vi "RSZVB Get Generator Step Attenuators.vi"(8 "error in (no error)":errorcluster {"code" format="%.0x"}, 9 "Port (1)":i32=1, 10 "Channel (1)":i32=1, 11 "VISA session":refnum<visa-resource-name>) -> (0 "error out":errorcluster {"code" format="%.0x"}, 1 "Attenuation Factor":dbl format="%^.3e", 3 "dup VISA session":refnum<visa-resource-name>)   [LabVIEW 2011]
doc: "This VI gets a fixed attenuation factor for the generated wave at test port no. <Pt>. \n\nNote(s):\n\n(1) This VI can be used only with R&S ZVA and ZVB instruments.\n\nRemote-control command(s):\nSOURce<Ch>:POWer<Pt>:ATTenuation?"
uses:
  _utility/RSZVB Global Data.vi
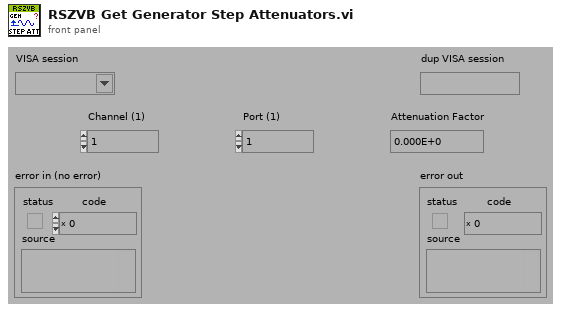
[diagram p1: front panel]
types:
  T1 = cluster{"Error Checking (T: On)":bool, "Installed Options":string[], "Data Valid?":bool, "Ports":i32, "Model":string[], "Option Checking (T: On)":bool}[]
  T2 = cluster{"Error Checking (T: On)":bool, "Installed Options":string[], "Data Valid?":bool, "Ports":i32, "Model":string[], "Option Checking (T: On)":bool}
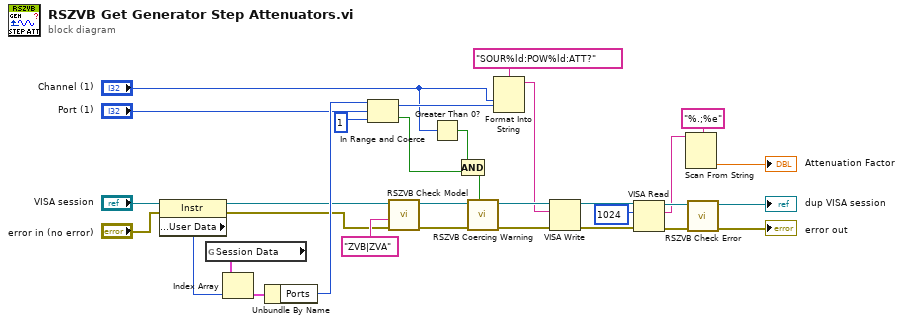
[diagram p0: block diagram]
diagram:
  n1 = property class="Instr"(reference="VISA session", error in="error in (no error)") -> (reference out=w19:refnum<visa-resource-name>, error out=w18:errorcluster, "General Settings:User Data"=w21:u32)
  n2 = global read "RSZVB Global Data.vi" "Session Data"() -> (w22:T1)
  n3 = Index Array(array=w22, index=w21) -> (element=w23:T2)
  n4 = Unbundle By Name(w23) -> ("Ports"=w20:i32)
  n5 = In Range and Coerce(upper limit=w20, x="Port (1)", lower limit=1) -> (coerced(x)=w16:i32, In Range?=w17:bool)
  n6 = call "RSZVB Check Model.vi"("error in (no error)"=w18, "Model"="ZVB|ZVA" ("Options"), "VISA session"=w19) -> ("error out"=w26:errorcluster, "dup VISA session"=w25:refnum<visa-resource-name>)  [unwired: 7 in]
  n7 = Greater Than 0?(x="Channel (1)") -> (x > 0?=w27:bool)
  n8 = Compound Arithmetic op=AND(w27, w17) -> (w29:bool)
  n9 = call "RSZVB Coercing Warning.vi"("In Range?"=w29, "error in (no error)"=w26, "VISA session"=w25) -> ("error out"=w30:errorcluster, "dup VISA session"=w31:refnum<visa-resource-name>)  [unwired: 7 in]
  n10 = Format Into String(format string="SOUR%ld:POW%ld:ATT?", "Channel (1)", w16) -> (resulting string=w28:string)  [unwired: 2 in, 1 out]
  n11 = VISA Write(VISA resource name=w31, write buffer=w28, error in (no error)=w30) -> (VISA resource name out=w5:refnum<visa-resource-name>, error out=w1:errorcluster)  [unwired: 1 out]
  n12 = VISA Read(VISA resource name=w5, byte count=u32 1024 ("byte count (0)"), error in (no error)=w1) -> (VISA resource name out=w9:refnum<visa-resource-name>, read buffer=w6:string, error out=w8:errorcluster)  [unwired: 1 out]
  n13 = Scan From String(format string="%.;%e", input string=w6) -> (output 1=→"Attenuation Factor":dbl)  [unwired: 3 in, 3 out]
  n14 = call "RSZVB Check Error.vi"("error in (no error)"=w8, "VISA session"=w9) -> ("error out"=→"error out":errorcluster, "dup VISA session"=→"dup VISA session":refnum<visa-resource-name>)  [unwired: 8 in]
